vi "avaiable tag menu action.vi"(8 "channel":refnum<class "TBM channel.lvclass">, 9 "selected tag":refnum<class "tag descriptor.lvclass">, 10 "action":T1, 11 "object ref":T2) -> (0 "error out":errorcluster, 2 "update?":bool)   [LabVIEW 2013, in "Table Manager.lvlib"]
uses:
  Table Manager.lvlib
  Table Manager/object ref.ctl
  Configuration Editor/Classes/Engine Parent/Engine Parent Editor Node.lvclass
  Configuration Editor/Classes/Module editor node/module editor node.lvclass
  <vilib>/NI/Tag Bus/tag/tag descriptor.lvclass
  <vilib>/NI/Tag Bus Module Framework/channel/TBM channel.lvclass
  control module/editor node/dialog output action.ctl
  <vilib>/NI/Configuration Framework/serializable configuration/NISE_CEF_serializable configuration.lvclass/NISE_CEF_serializable configuration.ctl
  <vilib>/Utility/LVClass/Get LV Class Name.vi
  <vilib>/NI/Configuration Framework/error generator/NISE_error generator.vi
  Configuration Editor/Classes/Module editor node/Read Module Configuration.vi
  <vilib>/NI/Tag Bus Module Framework/module configuration/TBM module configuration.lvclass
  <vilib>/NI/Module Execution Interface/Engine Configuration/engine configuration.lvclass
  <vilib>/NI/Configuration Framework/serializable configuration/NISE_CEF_serializable configuration.lvclass
  control module/editor node/control module editor.lvclass
  control module/configuration/control module configuration.lvclass
  Table Manager/Table Manager.lvclass
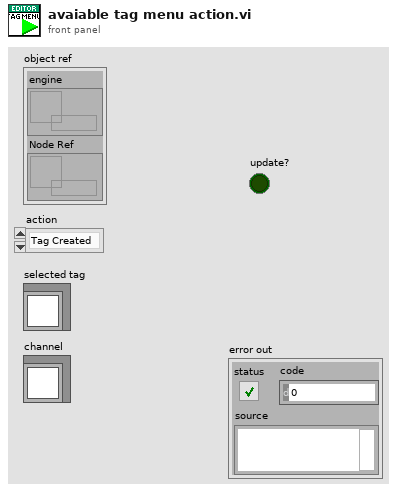
[diagram p1: front panel]
types:
  T1 = typedef "control module editor.lvclass/dialog output action.ctl" = enum16{"Tag Created", "Tag Selected", "Set Default", "disconnect"}
  T2 = typedef "Table Manager.lvlib/Table Manager.lvclass/object ref.ctl" = cluster{"engine":refnum<data-value>, "Node Ref":refnum<data-value>}
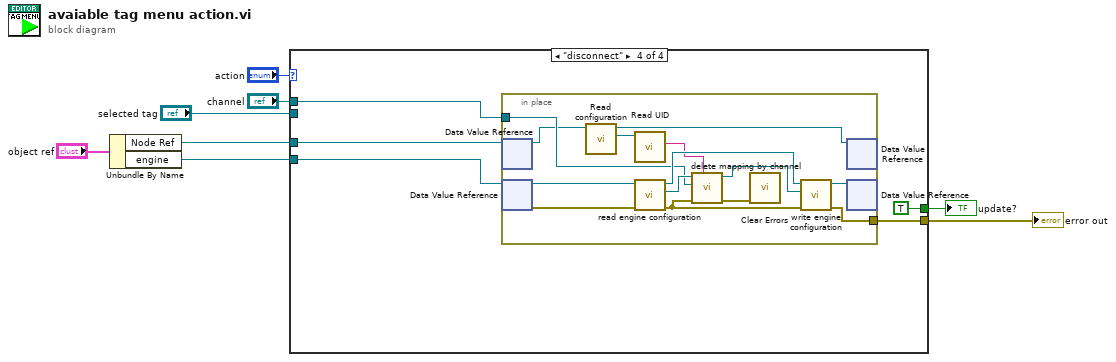
[diagram p0: block diagram]
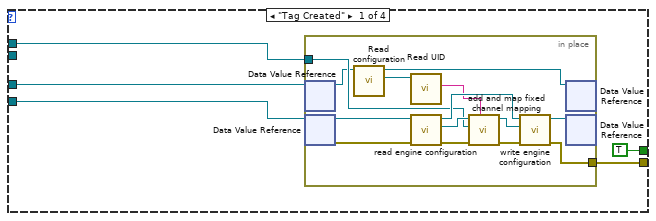
[diagram p2: hidden frame]
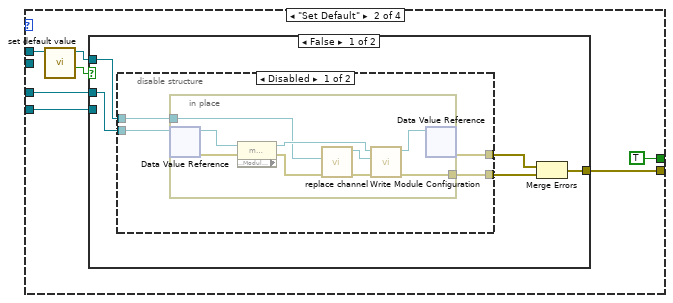
[diagram p3: hidden frame]
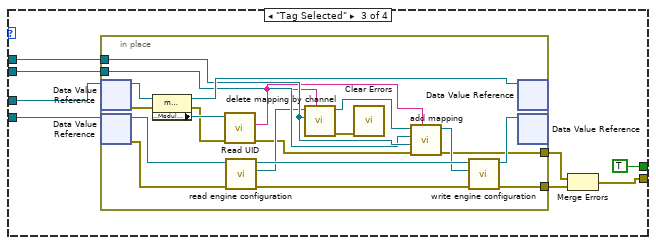
[diagram p6: hidden frame]
diagram:
  n1 = Unbundle By Name("object ref") -> ("Node Ref"=w6:refnum<data-value>, "engine"=w7:refnum<data-value>)
  n2 = case shown="\"disconnect\"" "action" {
    tunnel: "channel" -> [w13 w32 w60 w86]
    tunnel: "selected tag" -> [_ _ w56 _]
    tunnel: [w10 w34 w61 w84] -> w5
    tunnel: w6 -> [w11 w33 w55 w83]
    tunnel: w7 -> [w12 w29 w59 w85]
    tunnel: [TRUE ("update?") TRUE ("update?") TRUE ("update?") TRUE ("update?")] -> w1
    frame "Tag Created" {
      n3 = in-place {
        in-place-border: [w24] -> w10
        in-place-border: w13 -> [w20]
        n4 = in-place-dvr #1(w11) -> (w17:refnum<class "module editor node.lvclass">)  [unwired: 1 out]
        n5 = in-place-dvr #2(w12) -> (w26:refnum<class "Engine Parent Editor Node.lvclass">, w27:errorcluster)
        n6 = call-dynamic "Read configuration.vi"("NISE_CEF_serializable node in"=w17) -> ("configuration"=w15:refnum<class "NISE_CEF_serializable configuration.lvclass">, "NISE_CEF_serializable node out"=w16:refnum<class "module editor node.lvclass">)  [unwired: 8 in, 1 out]
        n7 = call <vilib>:"Read UID.vi"("configuration in"=w15) -> ("instance id"=w14:string)  [unwired: 8 in, 2 out]
        n8 = call "read engine configuration.vi"("error in"=w27, "Engine Parent Editor Node in"=w26) -> ("error out"=w19:errorcluster, "engine configuration"=w22:refnum<class "engine configuration.lvclass">, "Engine Parent Editor Node out"=w23:refnum<class "Engine Parent Editor Node.lvclass">)  [unwired: 7 in]
        n9 = call <vilib>:"add and map fixed channel mapping.vi"("module instance"=w14, "error in"=w19, "fixed channel"=w20, "engine configuration in"=w22) -> ("error out"=w18:errorcluster, "engine configuration out"=w21:refnum<class "engine configuration.lvclass">)  [unwired: 6 in]
        n10 = call "write engine configuration.vi"("error in"=w18, "engine configuration"=w21, "Engine Parent Editor Node in"=w23) -> ("error out"=w24:errorcluster, "Engine Parent Editor Node out"=w25:refnum<class "Engine Parent Editor Node.lvclass">)  [unwired: 7 in]
        n11 = in-place-dvr #1(w16) -> ()  [unwired: 2 out]
        n12 = in-place-dvr #2(w25) -> ()  [unwired: 2 out]
      }
    }
    frame "Set Default" {
      n13 = call "set default value.vi"("tag"=w32) -> ("cancelled?"=w30:bool, "tag out"=w31:refnum<class "TBM channel.lvclass">)  [unwired: 9 in]
      n14 = case shown="False" w30 {
        tunnel: [w37 _] -> w34
        tunnel: w33 -> [w39 _]
        tunnel: w31 -> [w38 _]
        tunnel: w29 -> [_ _]
        frame False {
          n15 = disable-structure shown="Disabled" {
            disable-tunnel: w39 -> [w43 _]
            disable-tunnel: w38 -> [w42 _]
            disable-tunnel: [w41 _] -> w36
            disable-tunnel: [w40 _] -> w35
            frame Disabled {
              n16 = in-place {
                in-place-border: w42 -> [w49]
                in-place-border: [w48] -> w40
                n17 = in-place-dvr #3(w43) -> (w51:refnum<class "module editor node.lvclass">, w47:errorcluster)
                n18 = property class="module editor node"(reference=w51, error in=w47) -> (reference out=w50:refnum<class "module editor node.lvclass">, error out=w46:errorcluster, "Data Access:Module Configuration"=w44:refnum<class "TBM module configuration.lvclass">)
                n19 = call "replace channel.vi"("error in"=w46, "channel"=w49) -> ("error out"=w45:errorcluster, "fixed module parent implementation configuration out"=w52:refnum<class "control module configuration.lvclass">)  [unwired: 8 in]
                n20 = call "Write Module Configuration.vi"("error in"=w45, "module configuration"=w52, "Module Editor Node in"=w50) -> ("error out"=w48:errorcluster, "Module Editor Node out"=w53:refnum<class "module editor node.lvclass">)  [unwired: 7 in]
                n21 = in-place-dvr #3(w53) -> (w41:errorcluster)  [unwired: 1 out]
              }
            }
            frame Enabled {
            }
          }
          n22 = Merge Errors(w36, w35) -> (w37:errorcluster)
        }
        frame True {
        }
      }
    }
    frame "Tag Selected" {
      n23 = in-place {
        in-place-border: [w71] -> w58
        in-place-border: w60 -> [w79]
        in-place-border: [w76] -> w57
        in-place-border: w56 -> [w70]
        n24 = in-place-dvr #4(w55) -> (w81:refnum<class "module editor node.lvclass">, w78:errorcluster)
        n25 = in-place-dvr #5(w59) -> (w74:refnum<class "Engine Parent Editor Node.lvclass">, w75:errorcluster)
        n26 = property class="module editor node"(reference=w81, error in=w78) -> (reference out=w80:refnum<class "module editor node.lvclass">, error out=w64:errorcluster, "Data Access:Module Configuration"=w66:refnum<class "TBM module configuration.lvclass">)
        n27 = call <vilib>:"Read UID.vi"("error in"=w64, "configuration in"=w66) -> ("error out"=w63:errorcluster, "instance id"=w67:string)  [unwired: 7 in, 1 out]
        n28 = call "read engine configuration.vi"("error in"=w75, "Engine Parent Editor Node in"=w74) -> ("error out"=w65:errorcluster, "engine configuration"=w69:refnum<class "engine configuration.lvclass">, "Engine Parent Editor Node out"=w73:refnum<class "Engine Parent Editor Node.lvclass">)  [unwired: 7 in]
        n29 = call <vilib>:"delete mapping by channel.vi"("owner ID"=w67, "channel"=w79, "engine configuration in"=w69) -> ("error out"=w62:errorcluster, "engine configuration out"=w68:refnum<class "engine configuration.lvclass">)  [unwired: 7 in]
        n30 = call <vilib>:"Clear Errors.vi"("error in (no error)"=w62) -> ()  [unwired: 6 in, 1 out]
        n31 = call <vilib>:"add mapping.vi"("owner ID"=w67, "error in"=w63, "channel"=w79, "tag descriptor"=w70, "engine configuration"=w68) -> ("error out"=w71:errorcluster, "engine configuration out"=w72:refnum<class "engine configuration.lvclass">)  [unwired: 5 in]
        n32 = call "write engine configuration.vi"("error in"=w65, "engine configuration"=w72, "Engine Parent Editor Node in"=w73) -> ("error out"=w76:errorcluster, "Engine Parent Editor Node out"=w77:refnum<class "Engine Parent Editor Node.lvclass">)  [unwired: 7 in]
        n33 = in-place-dvr #4(w80) -> ()  [unwired: 2 out]
        n34 = in-place-dvr #5(w77) -> ()  [unwired: 2 out]
      }
      n35 = Merge Errors(w58, w57) -> (w61:errorcluster)
    }
    frame "disconnect" {
      n36 = in-place {
        in-place-border: w86 -> [w92]
        in-place-border: [w97] -> w84
        n37 = in-place-dvr #6(w83) -> (w87:refnum<class "module editor node.lvclass">)  [unwired: 1 out]
        n38 = in-place-dvr #7(w85) -> (w100:refnum<class "Engine Parent Editor Node.lvclass">, w99:errorcluster)
        n39 = call-dynamic "Read configuration.vi"("NISE_CEF_serializable node in"=w87) -> ("configuration"=w90:refnum<class "NISE_CEF_serializable configuration.lvclass">, "NISE_CEF_serializable node out"=w88:refnum<class "module editor node.lvclass">)  [unwired: 8 in, 1 out]
        n40 = call <vilib>:"Read UID.vi"("configuration in"=w90) -> ("instance id"=w89:string)  [unwired: 8 in, 2 out]
        n41 = call "read engine configuration.vi"("error in"=w99, "Engine Parent Editor Node in"=w100) -> ("error out"=w94:errorcluster, "engine configuration"=w95:refnum<class "engine configuration.lvclass">, "Engine Parent Editor Node out"=w96:refnum<class "Engine Parent Editor Node.lvclass">)  [unwired: 7 in]
        n42 = call <vilib>:"delete mapping by channel.vi"("owner ID"=w89, "error in"=w94, "channel"=w92, "engine configuration in"=w95) -> ("error out"=w91:errorcluster, "engine configuration out"=w93:refnum<class "engine configuration.lvclass">)  [unwired: 6 in]
        n43 = call <vilib>:"Clear Errors.vi"("error in (no error)"=w91) -> ()  [unwired: 6 in, 1 out]
        n44 = call "write engine configuration.vi"("error in"=w94, "engine configuration"=w93, "Engine Parent Editor Node in"=w96) -> ("error out"=w97:errorcluster, "Engine Parent Editor Node out"=w98:refnum<class "Engine Parent Editor Node.lvclass">)  [unwired: 7 in]
        n45 = in-place-dvr #6(w88) -> ()  [unwired: 2 out]
        n46 = in-place-dvr #7(w98) -> ()  [unwired: 2 out]
      }
    }
  }
  "error out" <- w5
  "update?" <- w1
